vi "History Length Write.vi"(4 "error in (no error)":errorcluster, 5 "Value":i32, 6 "Container State":T2, 7 "Display State In":T1) -> (0 "error out":errorcluster, 3 "Display State Out":T1)   [LabVIEW 2009, in "HistoryPath.xctl"]
uses:
  HistoryPath.xctl
  <vilib>/_xctls/Container State.ctl
  State.ctl
  <vilib>/_xctls/XControlSupport.lvlib
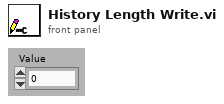
[diagram p1: front panel]
types:
  T1 = typedef "HistoryPath.xctl/State.ctl" = cluster{"History":path[], "History Length":i32}
  T2 = typedef "XControlSupport.lvlib/Container State.ctl" = cluster{"Indicator?":bool, "Run Mode?":bool, " Refnum":refnum<vi>}
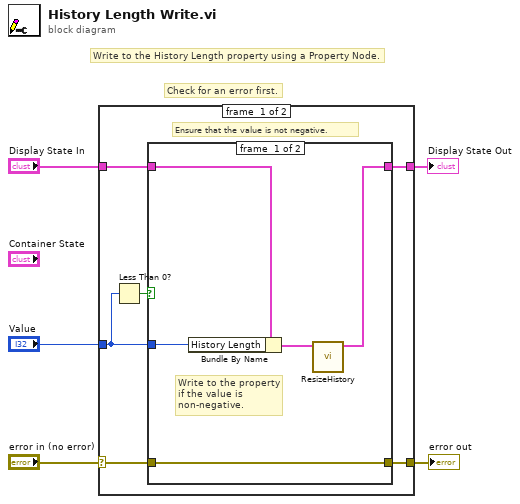
[diagram p0: block diagram]
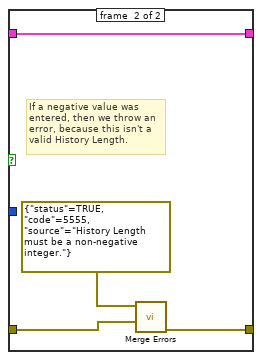
[diagram p2: hidden frame]
diagram:
  # "Check for an error first."
  # "Write to the History Length property using a Property Node."
  n1 = case shown="No Error" "error in (no error)" {
    selector: "error in (no error)" -> [w6 w21]
    tunnel: "Display State In" -> [w11 w22]
    tunnel: [w10 w22] -> w4
    tunnel: [w9 w21] -> w3
    tunnel: "Value" -> [w7 _]
    frame #0 {
      # "Ensure that the value is not negative."
      n2 = Less Than 0?(x=w7) -> (x < 0?=w8:bool)
      n3 = case shown="False" w8 {
        tunnel: w11 -> [w15 w20]
        tunnel: [w12 w20] -> w10
        tunnel: w6 -> [w16 w18]
        tunnel: [w16 w19] -> w9
        tunnel: w7 -> [w14 _]
        frame #0 {
          # "Write to the property\nif the value is\nnon-negative."
          n4 = Bundle By Name(cluster=w15, "History Length"=w14) -> (w13:T1)
          n5 = call "ResizeHistory.vi"("State In"=w13) -> ("State Out"=w12:T1)  [unwired: 10 in]
        }
        frame #1 {
          # "If a negative value was entered, then we throw an error, because this isn't a valid History Length."
          n6 = call <vilib>:"Merge Errors.vi"("error in 3 (no error)"=w18, "error in 1 (no error)"=errorcluster {"status"=TRUE, "code"=5555, "source"="History Length must be a non-negative integer."}) -> ("error out"=w19:errorcluster)  [unwired: 5 in]
        }
      }
    }
    frame #1 {
    }
  }
  "error out" <- w3
  "Display State Out" <- w4
